vi "AddLabelsInSetupGroup.vi"(0 "Engine In":refnum<k7>, 5 "SequenceFile In":refnum<k7>, 11 "Error In":errorcluster) -> (4 "Engine Out":refnum<k7>, 6 "SequenceFile Out":refnum<k7>, 15 "Error Out":errorcluster)   [LabVIEW 2021, in "Create Sequence.lvlib"]
doc: "Adds the required instruction steps on the 'SetupGroup'"
uses:
  Create Sequence.lvlib
  TypeDef/StepProperties.ctl
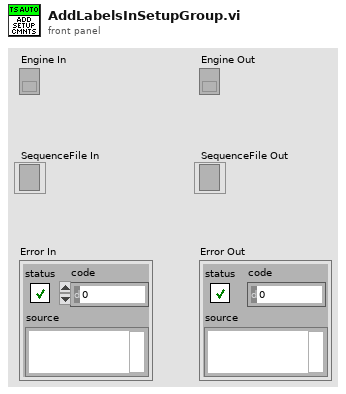
[diagram p1: front panel]
types:
  T1 = typedef "Create Sequence.lvlib/StepProperties.ctl" = cluster{"StepTypeName":string, "StepName":string, "Description":string, "Comment":string, "sequenceNameParam":string, "Step Group":i32, "Step Index":i32, "Expression":string}
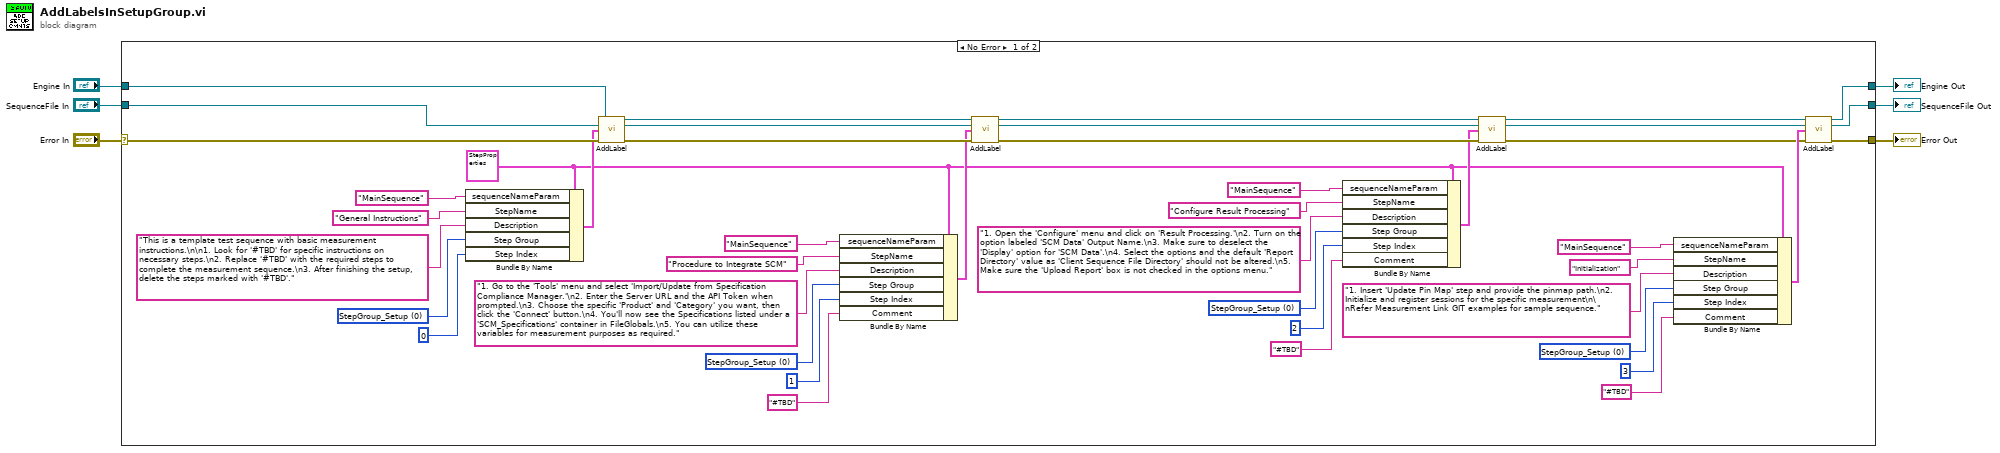
[diagram p0: block diagram]
diagram:
  n1 = case shown="No Error" "Error In" {
    selector: "Error In" -> [w43 w52]
    tunnel: "Engine In" -> [w39 w50]
    tunnel: "SequenceFile In" -> [w41 w51]
    tunnel: [w46 w50] -> w3
    tunnel: [w45 w51] -> w2
    tunnel: [w44 w52] -> w1
    frame No Error {
      w13 = 0 items=["StepGroup_Setup", "StepGroup_Main", "StepGroup_Cleanup"] ("Step Group")
      w23 = 0 items=["StepGroup_Setup", "StepGroup_Main", "StepGroup_Cleanup"] ("Step Group")
      w26 = 0 items=["StepGroup_Setup", "StepGroup_Main", "StepGroup_Cleanup"] ("Step Group")
      w11 = T1 {"StepTypeName"="", "StepName"="", "Description"="", "Comment"="", "sequenceNameParam"="MainSequence", "Step Group"=0, "Step Index"=3, "Expression"=""} ("StepProperties")
      w34 = 0 items=["StepGroup_Setup", "StepGroup_Main", "StepGroup_Cleanup"] ("Step Group")
      n2 = Bundle By Name(cluster=w11, "sequenceNameParam"="MainSequence", "StepName"="General Instructions" ("Step Name"), "Description"="This is a template test sequence with basic measurement instructions.\n\n1. Look for '#TBD' for specific instructions on necessary steps.\n2. Replace '#TBD' with the required steps to complete the measurement sequence.\n3. After finishing the setup, delete the steps marked with '#TBD'.", "Step Group"=w34, "Step Index"=0) -> (w32:T1)
      n3 = call "AddLabel.vi"("Engine In"=w39, "SequenceFile In"=w41, "StepProperties"=w32, "Error In"=w43) -> ("Engine Out"=w38:refnum<k7>, "SequenceFile Out"=w40:refnum<k7>, "Error Out"=w42:errorcluster)  [unwired: 9 in]
      n4 = Bundle By Name(cluster=w11, "sequenceNameParam"="MainSequence", "StepName"="Procedure to Integrate SCM" ("Step Name"), "Description"="1. Go to the 'Tools' menu and select 'Import/Update from Specification Compliance Manager.'\n2. Enter the Server URL and the API Token when prompted.\n3. Choose the specific 'Product' and 'Category' you want, then click the 'Connect' button.\n4. You'll now see the Specifications listed under a 'SCM_Specifications' container in FileGlobals.\n5. You can utilize these variables for measurement purposes as required.", "Step Group"=w26, "Step Index"=1, "Comment"="#TBD") -> (w31:T1)
      n5 = call "AddLabel.vi"("Engine In"=w38, "SequenceFile In"=w40, "StepProperties"=w31, "Error In"=w42) -> ("Engine Out"=w47:refnum<k7>, "SequenceFile Out"=w48:refnum<k7>, "Error Out"=w49:errorcluster)  [unwired: 9 in]
      n6 = Bundle By Name(cluster=w11, "sequenceNameParam"="MainSequence", "StepName"="Configure Result Processing" ("Step Name"), "Description"="1. Open the 'Configure' menu and click on 'Result Processing.'\n2. Turn on the option labeled 'SCM Data' Output Name.\n3. Make sure to deselect the 'Display' option for 'SCM Data'.\n4. Select the options and the default 'Report Directory' value as 'Client Sequence File Directory' should not be altered.\n5. Make sure the 'Upload Report' box is not checked in the options menu.", "Step Group"=w23, "Step Index"=2, "Comment"="#TBD") -> (w18:T1)
      n7 = call "AddLabel.vi"("Engine In"=w47, "SequenceFile In"=w48, "StepProperties"=w18, "Error In"=w49) -> ("Engine Out"=w9:refnum<k7>, "SequenceFile Out"=w8:refnum<k7>, "Error Out"=w7:errorcluster)  [unwired: 9 in]
      n8 = Bundle By Name(cluster=w11, "sequenceNameParam"="MainSequence", "StepName"="Initialization" ("Step Name"), "Description"="1. Insert 'Update Pin Map' step and provide the pinmap path.\n2. Initialize and register sessions for the specific measurement\n\nRefer Measurement Link GIT examples for sample sequence.", "Step Group"=w13, "Step Index"=3, "Comment"="#TBD") -> (w10:T1)
      n9 = call "AddLabel.vi"("Engine In"=w9, "SequenceFile In"=w8, "StepProperties"=w10, "Error In"=w7) -> ("Engine Out"=w46:refnum<k7>, "SequenceFile Out"=w45:refnum<k7>, "Error Out"=w44:errorcluster)  [unwired: 9 in]
    }
    frame Error {
    }
  }
  "Error Out" <- w1
  "Engine Out" <- w3
  "SequenceFile Out" <- w2
